vi "get_volume_issues.vi"(10 "id":i32[](array[numeric]), 11 "CV Comics in":refnum<class "CV Comics.lvclass">) -> (1 "issues":string[][](array[string]), 2 "names":string[](array[string]), 3 "CV Comics out":refnum<class "CV Comics.lvclass">)   [LabVIEW 2024, in "CLZ_to_ComicVine.lvlib" / "CV Comics.lvclass"]
uses:
  CV Comics.lvclass
  CV Comics.lvclass/CV Comics.ctl
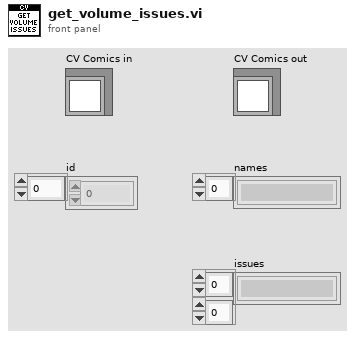
[diagram p1: front panel]
types:
  T1 = typedef "CLZ_to_ComicVine.lvlib/CV Comics.lvclass/volume--cluster.ctl" = cluster{"id":i32, "name":string, "issue set":set{cluster{string, string}}, "matched":bool}
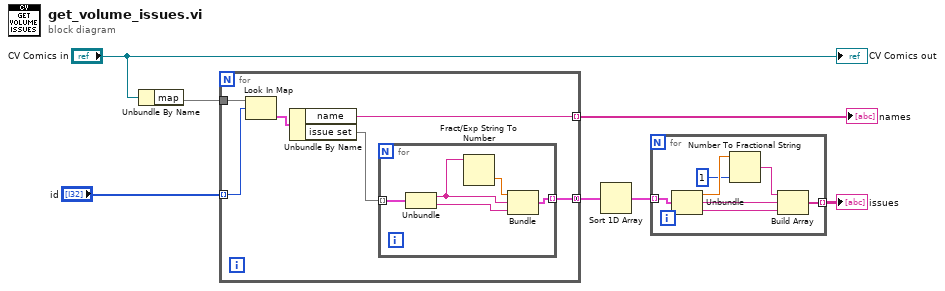
[diagram p0: block diagram]
diagram:
  n1 = Unbundle By Name("CV Comics in") -> ("map"=w6:map{i32, T1})
  n2 = for {
    tunnel: w6 -> [w13]
    tunnel: "id" -> [w12] mode=indexing
    tunnel: [w10] -> w4 mode=indexing
    tunnel: [w8] -> w3 mode=concatenating
    n3 = Look In Map(map=w13, key=w12) -> (value=w11:T1)  [unwired: 1 in, 1 out]
    n4 = Unbundle By Name(w11) -> ("name"=w10:string, "issue set"=w9:set{cluster{string, string}})
    n5 = for {
      tunnel: w9 -> [w16] mode=indexing
      tunnel: [w17] -> w8 mode=indexing
      n6 = Unbundle(w16) -> (w15:string, w14:string)
      n7 = Fract/Exp String To Number(string=w15) -> (number=w18:dbl)  [unwired: 3 in, 1 out]
      n8 = Bundle(w18, w15, w14) -> (w17:cluster{dbl, string, string})  [unwired: 1 in]
    }
  }
  "names" <- w4
  n9 = Sort 1D Array(array=w3) -> (sorted array=w2:cluster{dbl, string, string}[])
  n10 = for {
    tunnel: w2 -> [w25] mode=indexing
    tunnel: [w20] -> w1 mode=indexing
    n11 = Unbundle(w25) -> (w24:dbl, w22:string, w19:string)
    n12 = Number To Fractional String(number=w24, precision (6)=i16 1) -> (F-format string=w21:string)  [unwired: 2 in]
    n13 = Build Array(w21, w22, w19) -> (w20:string[])
  }
  "issues" <- w1
  "CV Comics out" <- "CV Comics in"
